vi "ArrayAsStrings.vi"(8 "error in (no error)":errorcluster, 11 "Array Parameter":string="\n      <array>\n  <data>\r<value><string>0.000000</string></value>\r<value><string>1.175571</string></value>\r<value><string>1.902113</string></value>\r\n</data>\n</array>\n    ") -> (0 "error out":errorcluster, 3 "ArrayAsStrings":string[](array[string]))   [LabVIEW 2009]
doc: "Convert an XML-RPC formatted array of strings to a LV array of strings"
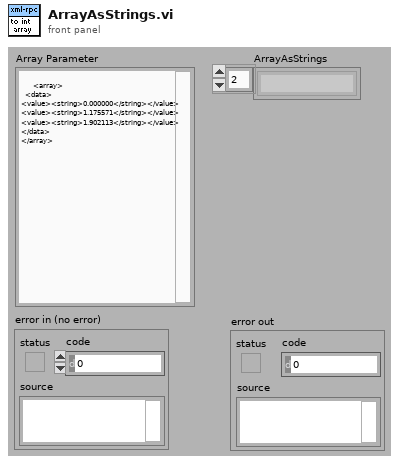
[diagram p1: front panel]
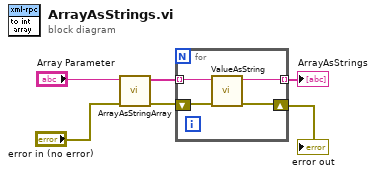
[diagram p0: block diagram]
diagram:
  n1 = call "ArrayAsStringArray.vi"("error in (no error)"="error in (no error)", "Array Parameter"="Array Parameter") -> ("error out"=w3:errorcluster, "ArrayAsValues"=w4:string[])  [unwired: 8 in]
  n2 = for {
    tunnel: w4 -> [w10] mode=indexing
    shift-right: [w8] -> w2
    shift-left: w3 -> [w9]
    tunnel: [w7] -> w1 mode=indexing
    n3 = call "ValueAsString.vi"("error in (no error)"=w9, "Parameter"=w10) -> ("error out"=w8:errorcluster, "value"=w7:string)  [unwired: 8 in]
  }
  "ArrayAsStrings" <- w1
  "error out" <- w2
